vi "Add Line.vi"(8 "error in":errorcluster, 10 "Line":T1, 11 "Benchmark PID configuration in":refnum<class "Benchmark PID configuration.lvclass">) -> (0 "error out":errorcluster, 2 "Line Index":i32, 3 "Benchmark PID configuration out":refnum<class "Benchmark PID configuration.lvclass">)   [LabVIEW 2018, in "Benchmark PID configuration.lvclass"]
doc: "Adds a new line to a configuration."
uses:
  Benchmark PID configuration.lvclass
  <vilib>/NI/Tag Bus Module Framework/channel/TBM channel.lvclass
  Line.ctl
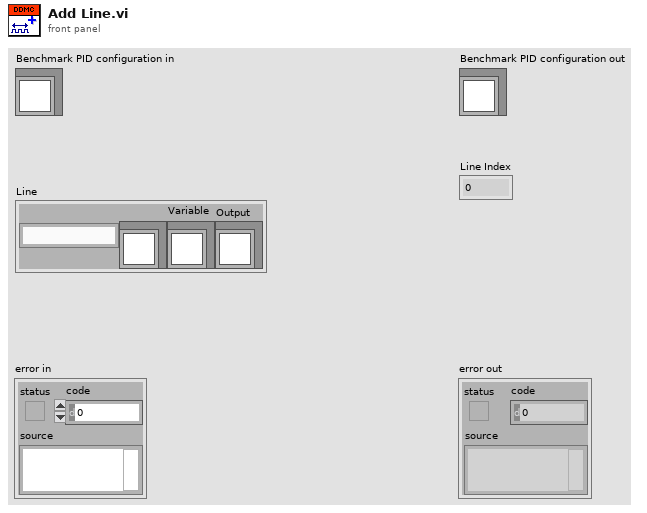
[diagram p1: front panel]
types:
  T1 = typedef "Benchmark PID configuration.lvclass/Line.ctl" = cluster{"PID Name":string, "Setpoint":refnum<class "TBM channel.lvclass">, "Variable":refnum<class "TBM channel.lvclass">, "Output":refnum<class "TBM channel.lvclass">}
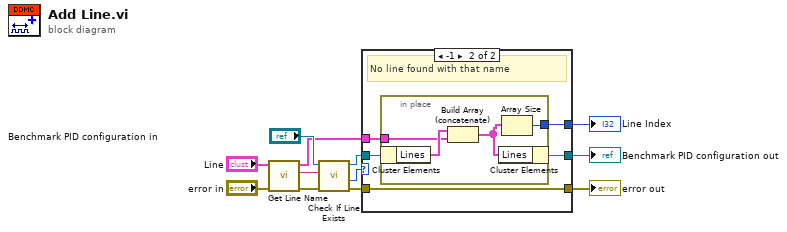
[diagram p0: block diagram]
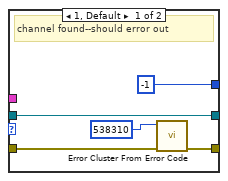
[diagram p2: hidden frame]
diagram:
  n1 = call "Get Line Name.vi"("error in"="error in", "Line in"="Line") -> ("error out"=w7:errorcluster, "Name"=w6:string, "Line out"=w4:T1)  [unwired: 7 in]
  n2 = call-dynamic "Check If Line Exists.vi"("error in"=w7, "Name to Locate"=w6, "Benchmark PID configuration in"="Benchmark PID configuration in") -> ("error out"=w8:errorcluster, "Index"=w3:i32, "Benchmark PID configuration out"=w2:refnum<class "Benchmark PID configuration.lvclass">)  [unwired: 4 in, 2 out]
  n3 = case shown="-1" w3 {
    tunnel: [w17 w21] -> w12
    tunnel: w8 -> [w15 w21]
    tunnel: w2 -> [w14 w20]
    tunnel: w4 -> [_ w22]
    tunnel: [w14 w19] -> w11
    tunnel: [-1 w18] -> w1
    frame 1, Default {
      # "channel found--should error out"
      n4 = call <vilib>:"Error Cluster From Error Code.vi"("error in (no error)"=w15, "error code (0)"=538310) -> ("error out"=w17:errorcluster)  [unwired: 7 in]
    }
    frame -1 {
      # "No line found with that name"
      n5 = in-place {
        in-place-border: w22 -> [w25]
        in-place-border: [w23] -> w18
        n6 = in-place-cluster #1(w20) -> ("Lines"=w26:T1[])
        n7 = Build Array (concatenate)(w26, w25) -> (w24:T1[])
        n8 = in-place-cluster #1("Lines"=w24) -> (w19:refnum<class "Benchmark PID configuration.lvclass">)
        n9 = Array Size(array=w24) -> (size(s)=w23:i32)
      }
    }
  }
  "error out" <- w12
  "Benchmark PID configuration out" <- w11
  "Line Index" <- w1
